vi "RVC Create Serial Arm.vi"() -> ()   [LabVIEW 2013]
uses:
  <vilib>/robotics/Kinematics/Analytical/SCARA/Initialize SCARA Serial Arm.vi
  <vilib>/robotics/Kinematics/Analytical/Initialize Generic Serial Arm.vi
  <vilib>/robotics/Kinematics/Analytical/NI_Robotics_AnalyticKinematics.lvlib
  <vilib>/robotics/Kinematics/Robot/NI_Robotics_Serial Robot Arm.lvclass
  <vilib>/robotics/Kinematics/Link/Joint Type.ctl
  <vilib>/robotics/Kinematics/Link/NI_Robotics_Link.lvclass
  <vilib>/robotics/Kinematics/DH Kinematic Parameters.ctl
  <vilib>/robotics/Kinematics/NI_Kinematics.lvlib
  <vilib>/robotics/Kinematics/Analytical/SCARA/NI_Robotics_SCARA Serial Arm Class.lvclass
panel:
  out "Scara":refnum<vi>(3d-picture)
  out "L.A (.0.5)":picture
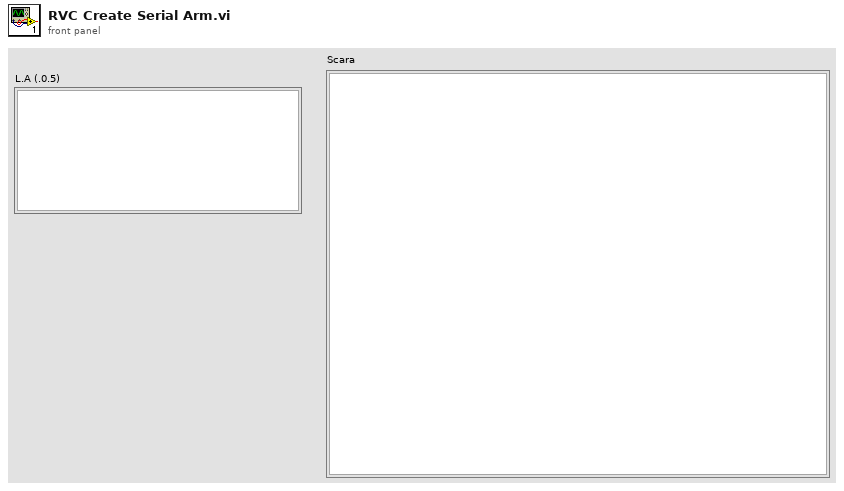
[diagram p1: front panel]
types:
  T1 = typedef "DH Kinematic Parameters.ctl" = cluster{"twist angle":dbl, "length":dbl, "rotation angle":dbl, "offset distance":dbl, "joint type":T2, "joint coordinate offset":dbl}
  T2 = typedef "NI_Robotics_Link.lvclass/Joint Type.ctl" = enum16{"Revolute", "Prismatic"}
  T3 = typedef "NI_Matrix.lvlib/RealMatrix.ctl" = dbl[][]
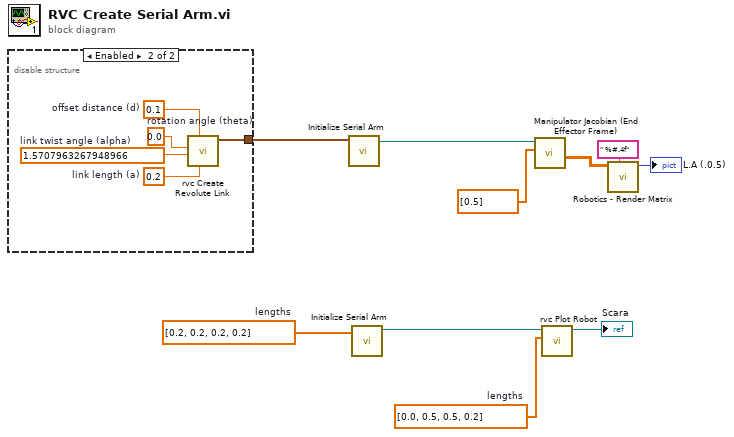
[diagram p0: block diagram]
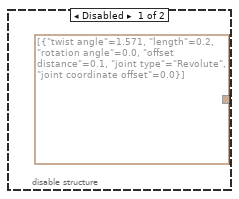
[diagram p2: hidden frame]
diagram:
  w1 = dbl[] [0.0, 0.5, 0.5, 0.2]  # lengths
  w2 = dbl[] [0.2, 0.2, 0.2, 0.2]  # lengths
  n1 = disable-structure shown="Enabled" {
    disable-tunnel: [T1[] [{"twist angle"=1.571, "length"=0.2, "rotation angle"=0.0, "offset distance"=0.1, "joint type"=enum."Revolute", "joint coordinate offset"=0.0}] ("kinematic parameters") w16] -> w6
    frame Disabled {
    }
    frame Enabled {
      w12 = 1.5707963267948966  # link twist angle (alpha)
      w13 = 0.1  # offset distance (d)
      w14 = 0.2  # link length (a)
      w15 = 0.0  # rotation angle (theta)
      n2 = call "rvc Create Revolute Link.vi"("length (a)"=w14, "offset distance (d)"=w13, "twist angle (alpha)"=w12, "rotation angle (theta)"=w15) -> ("Array"=w16:T1[])  [unwired: 7 in]
    }
  }
  n3 = call-poly <vilib>:"Initialize Serial Arm.vi"("kinematic parameters"=w6) -> ("serial arm out"=w7:refnum<class "NI_Robotics_Serial Robot Arm.lvclass">)  [unwired: 9 in, 1 out]
  n4 = call-poly <vilib>:"Initialize Serial Arm.vi"("lengths"=w2) -> ("SCARA serial arm out"=w4:refnum<class "NI_Robotics_SCARA Serial Arm Class.lvclass">)  [unwired: 9 in, 1 out]
  n5 = call <vilib>:"Manipulator Jacobian (End Effector Frame).vi"("joint positions"=dbl[] [0.5], "serial arm in"=w7) -> ("forward kinematics"=w8:T3)  [unwired: 6 in, 3 out]
  n6 = call "rvc Plot Robot.vi"("joint positions"=w1, "NI_Robotics_Serial Robot Arm in"=w4) -> ("Scene Object Out"=→"Scara":refnum<vi>)  [unwired: 8 in, 1 out]
  n7 = call "Robotics - Render Matrix.vi"("format string"=" %#.4f", "A"=w8) -> ("picture out"=→"L.A (.0.5)":picture)  [unwired: 9 in]
